vi "Benchmark Delete With Type Check.vi"() -> ()   [LabVIEW 2017]
uses:
  Source/LookupTable/LookupTable.lvclass/LookupTable.ctl
  3f600695-5b5a-4146-a4af-1e267d96d976.vi
  b6b64ea5-f314-4d4f-8fa7-59ac42c8a07d.vi
  Source/LookupTable/Read Table Reference.vi
  Source/LookupTable/LookupTable.lvclass
panel:
  in  "Table Size":i32=100000
  out "Variant DVR":dbl
  out "Waveform Chart":cluster{dbl, dbl, dbl}(graph)
  out "Variant by value":dbl
  out "Composed Lookup Table":dbl
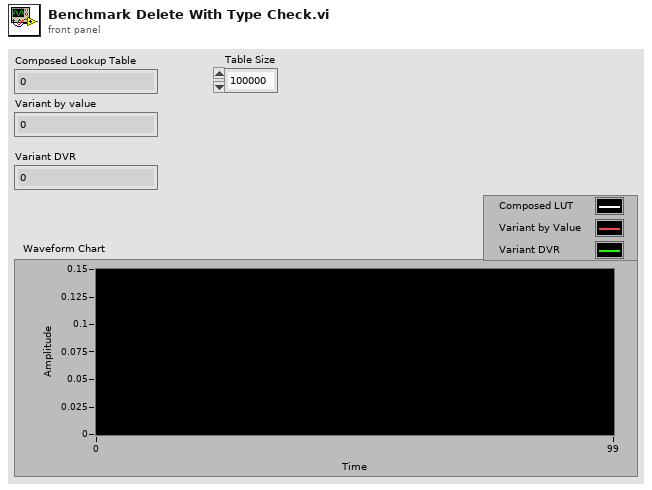
[diagram p1: front panel]
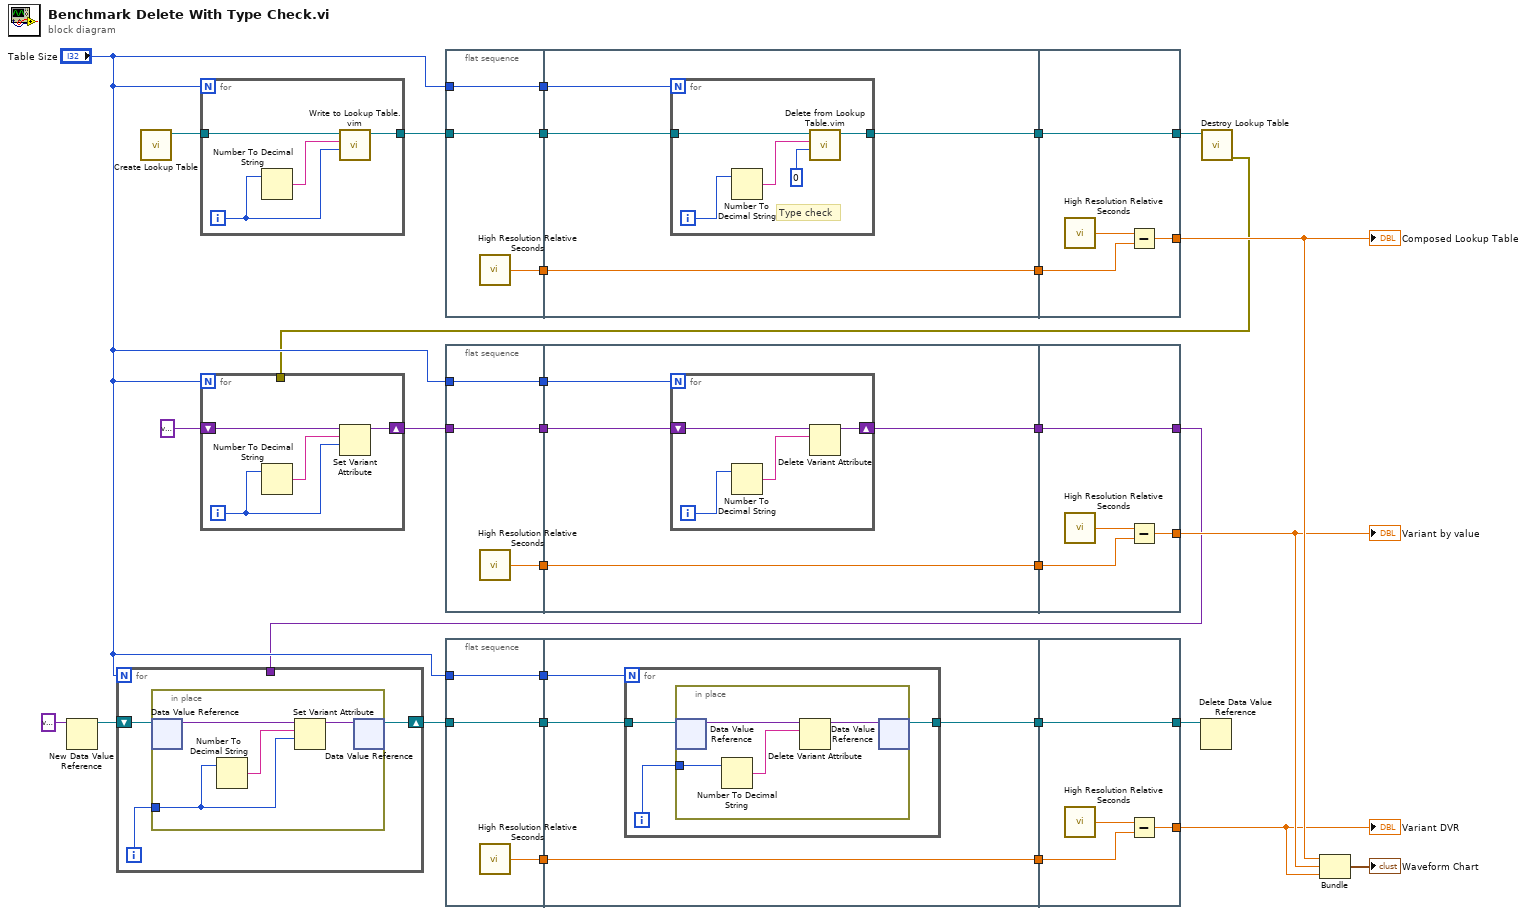
[diagram p0: block diagram]
diagram:
  n1 = New Data Value Reference(data value=variant) -> (data value reference=w12:refnum<data-value>)  [unwired: 1 in, 1 out]
  n2 = for {
    N: "Table Size" -> [_]
    shift-right: [w33] -> w11
    shift-left: w12 -> [w34]
    tunnel: w1 -> [_]
    i -> [w32]
    n3 = in-place {
      in-place-border: w32 -> [w35]
      n4 = in-place-dvr #1(w34) -> (w37:variant)  [unwired: 1 out]
      n5 = Number To Decimal String(number=w35) -> (decimal integer string=w38:string)  [unwired: 1 in]
      n6 = Set Variant Attribute(Variant=w37, name=w38, value=w35) -> (Variant out=w36:variant)  [unwired: 1 in, 2 out]
      n7 = in-place-dvr #1(w36) -> (w33:refnum<data-value>)  [unwired: 1 out]
    }
  }
  n8 = call "Create Lookup Table.vi"() -> ("LookupTable Reference"=w26:refnum<data-value>)  [unwired: 10 in, 1 out]
  n9 = for {
    N: "Table Size" -> [_]
    tunnel: [w40] -> w24
    tunnel: w26 -> [w39]
    i -> [w41]
    n10 = Number To Decimal String(number=w41) -> (decimal integer string=w42:string)  [unwired: 1 in]
    n11 = call "Write to Lookup Table.vim"("Item"=w41, "Item Name"=w42, "LookupTable Reference"=w39) -> ("LookupTable Reference Out"=w40:refnum<data-value>)  [unwired: 6 in, 2 out]
  }
  n12 = flat-sequence {
    tunnel: [w45] -> w31
    tunnel: [w44] -> w25
    tunnel: w24 -> [w44]
    tunnel: [w43] -> w19
    tunnel: "Table Size" -> [w43]
    tunnel: w31 -> [w49]
    tunnel: [w49] -> w30
    tunnel: w25 -> [w48]
    tunnel: [w47] -> w22
    tunnel: w19 -> [w46]
    tunnel: w30 -> [w57]
    tunnel: [w56] -> w9
    tunnel: [w55] -> w23
    tunnel: w22 -> [w55]
    frame #0 {
      n13 = call <vilib>:"High Resolution Relative Seconds.vi"() -> ("relative seconds"=w45:dbl)
    }
    frame #1 {
      n14 = for {
        N: w46 -> [_]
        tunnel: [w52] -> w47
        tunnel: w48 -> [w51]
        i -> [w53]
        # "Type check"
        n15 = Number To Decimal String(number=w53) -> (decimal integer string=w54:string)  [unwired: 1 in]
        n16 = call "Delete from Lookup Table.vim"("Confirm Type"=0, "Item Name"=w54, "LookupTable Reference"=w51) -> ("LookupTable Reference Out"=w52:refnum<data-value>)  [unwired: 6 in, 2 out]
      }
    }
    frame #2 {
      n17 = call <vilib>:"High Resolution Relative Seconds.vi"() -> ("relative seconds"=w58:dbl)
      n18 = Subtract(x=w58, y=w57) -> (x-y=w56:dbl)
    }
  }
  n19 = flat-sequence {
    tunnel: [w61] -> w29
    tunnel: [w60] -> w21
    tunnel: w20 -> [w60]
    tunnel: "Table Size" -> [w59]
    tunnel: [w59] -> w18
    tunnel: w29 -> [w65]
    tunnel: [w65] -> w28
    tunnel: w21 -> [w64]
    tunnel: w18 -> [w63]
    tunnel: [w62] -> w3
    tunnel: w28 -> [w72]
    tunnel: [w71] -> w8
    tunnel: [w70] -> w1
    tunnel: w3 -> [w70]
    frame #0 {
      n20 = call <vilib>:"High Resolution Relative Seconds.vi"() -> ("relative seconds"=w61:dbl)
    }
    frame #1 {
      n21 = for {
        N: w63 -> [_]
        shift-right: [w69] -> w62
        shift-left: w64 -> [w66]
        i -> [w67]
        n22 = Number To Decimal String(number=w67) -> (decimal integer string=w68:string)  [unwired: 1 in]
        n23 = Delete Variant Attribute(6:w68, 7:w66) -> (3:w69:variant)  [unwired: 1 in, 2 out]
      }
    }
    frame #2 {
      n24 = call <vilib>:"High Resolution Relative Seconds.vi"() -> ("relative seconds"=w73:dbl)
      n25 = Subtract(x=w73, y=w72) -> (x-y=w71:dbl)
    }
  }
  n26 = flat-sequence {
    tunnel: [w76] -> w17
    tunnel: [w75] -> w16
    tunnel: w11 -> [w75]
    tunnel: "Table Size" -> [w74]
    tunnel: [w74] -> w15
    tunnel: w17 -> [w80]
    tunnel: [w80] -> w14
    tunnel: w16 -> [w79]
    tunnel: w15 -> [w77]
    tunnel: [w78] -> w4
    tunnel: w14 -> [w90]
    tunnel: [w89] -> w7
    tunnel: [w88] -> w5
    tunnel: w4 -> [w88]
    frame #0 {
      n27 = call <vilib>:"High Resolution Relative Seconds.vi"() -> ("relative seconds"=w76:dbl)
    }
    frame #1 {
      n28 = for {
        N: w77 -> [_]
        tunnel: [w82] -> w78
        tunnel: w79 -> [w81]
        i -> [w83]
        n29 = in-place {
          in-place-border: w83 -> [w86]
          n30 = in-place-dvr #2(w81) -> (w85:variant)  [unwired: 1 out]
          n31 = Number To Decimal String(number=w86) -> (decimal integer string=w87:string)  [unwired: 1 in]
          n32 = Delete Variant Attribute(6:w87, 7:w85) -> (3:w84:variant)  [unwired: 1 in, 2 out]
          n33 = in-place-dvr #2(w84) -> (w82:refnum<data-value>)  [unwired: 1 out]
        }
      }
    }
    frame #2 {
      n34 = call <vilib>:"High Resolution Relative Seconds.vi"() -> ("relative seconds"=w91:dbl)
      n35 = Subtract(x=w91, y=w90) -> (x-y=w89:dbl)
    }
  }
  n36 = Delete Data Value Reference(data value reference=w5) -> ()  [unwired: 1 in, 2 out]
  n37 = call "Destroy Lookup Table.vi"("LookupTable Reference"=w23) -> ("error out"=w2:errorcluster)  [unwired: 10 in]
  n38 = for {
    N: "Table Size" -> [_]
    shift-right: [w95] -> w20
    shift-left: variant -> [w92]
    tunnel: w2 -> [_]
    i -> [w93]
    n39 = Number To Decimal String(number=w93) -> (decimal integer string=w94:string)  [unwired: 1 in]
    n40 = Set Variant Attribute(Variant=w92, name=w94, value=w93) -> (Variant out=w95:variant)  [unwired: 1 in, 2 out]
  }
  n41 = Bundle(w9, w8, w7) -> (→"Waveform Chart":cluster{dbl, dbl, dbl})  [unwired: 1 in]
  "Composed Lookup Table" <- w9
  "Variant by value" <- w8
  "Variant DVR" <- w7
